vi "Destroy Model.vi"(0 "Serial port asssistant model in":refnum<class "Serial port assistant model.lvclass">, 11 "error in (no error)":errorcluster) -> (4 "Serial port asssistant model out":refnum<class "Serial port assistant model.lvclass">, 15 "error out":errorcluster)   [LabVIEW 2022 SP3, in "Serial port assistant model.lvlib" / "Serial port assistant model.lvclass"]
uses:
  Serial port assistant model.lvclass
  Serial port assistant model.lvclass/Serial port assistant model.ctl
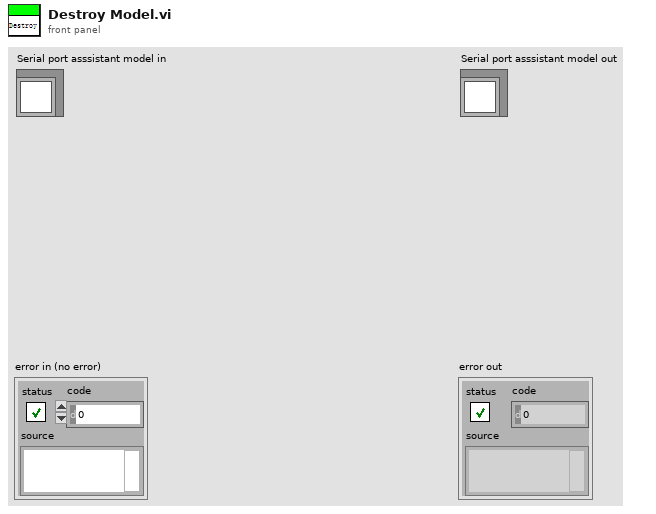
[diagram p1: front panel]
types:
  T1 = typedef "Rendezvous RefNum" = refnum<k1>
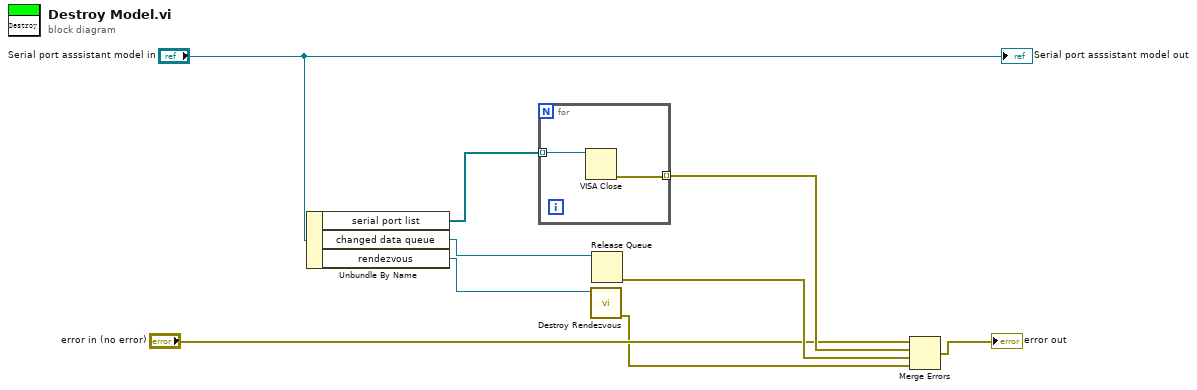
[diagram p0: block diagram]
diagram:
  n1 = Unbundle By Name("Serial port asssistant model in") -> ("serial port list"=w8:refnum<visa-resource-name>[], "changed data queue"=w6:refnum<queue>, "rendezvous"=w2:T1)
  n2 = for {
    tunnel: w8 -> [w11] mode=indexing
    tunnel: [w10] -> w7 mode=indexing
    n3 = VISA Close(VISA resource name=w11) -> (error out=w10:errorcluster)  [unwired: 1 in]
  }
  n4 = call <vilib>:"Destroy Rendezvous.vi"("rendezvous"=w2) -> ("error out"=w1:errorcluster)  [unwired: 5 in, 1 out]
  n5 = Release Queue(queue=w6) -> (error out=w5:errorcluster)  [unwired: 2 in, 2 out]
  n6 = Merge Errors("error in (no error)", w7, w5, w1) -> (→"error out":errorcluster)
  "Serial port asssistant model out" <- "Serial port asssistant model in"
